vi "Configure Digital Channel.vi"(7 "channel enabled (True)":bool=TRUE caption="Channel Enabled (True)", 8 "error in (no error)":errorcluster {"code" format="%.0x"}, 9 "input impedance (100.0E+3 ohms)":dbl=100000.0 caption="Input Impedance (100.0E+3 ohms)" format="%^.2e", 10 "Digital Channel (\"D0\")":string(combo)="DIG0", 11 "VISA Resource Name":refnum<visa-resource-name>) -> (0 "error out":errorcluster {"code" format="%.0x"}, 3 "VISA Resource Name Out":refnum<visa-resource-name>)   [LabVIEW 2011, in "Agilent 546XX Series.lvlib"]
doc: "This VI configures the common properties of the oscilloscope's digital channel subsystem for a specified digital channel. These properties are the input impedance and channel enabled.\n\nNOTES: \n\n(1) This VI is only supported by AG546xx\"D\" models. \n\n(2) This VI is only valid for digital channels."
uses:
  Agilent 546XX Series.lvlib
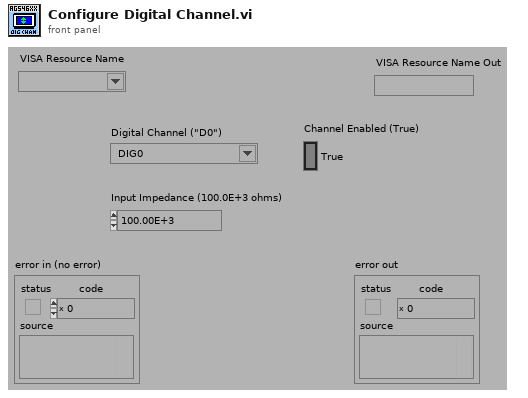
[diagram p1: front panel]
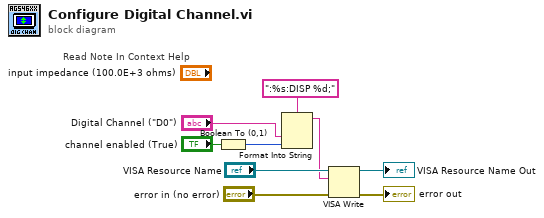
[diagram p0: block diagram]
diagram:
  # "Read Note In Context Help"
  n1 = Boolean To (0,1)(Boolean="channel enabled (True)") -> (0, 1=w2:i16)
  n2 = Format Into String(format string=":%s:DISP %d;", "Digital Channel (\"D0\")", w2) -> (resulting string=w1:string)  [unwired: 2 in, 1 out]
  n3 = VISA Write(VISA resource name="VISA Resource Name", write buffer=w1, error in (no error)="error in (no error)") -> (VISA resource name out=→"VISA Resource Name Out":refnum<visa-resource-name>, error out=→"error out":errorcluster)  [unwired: 1 out]
